vi "Prev_DaQ_QMH.vi"(8 "Error In":errorcluster, 11 "Queue In":refnum<queue>) -> (0 "Error Out":errorcluster, 1 "Message":variant, 2 "Instruction":T1=enum."Start DaQ", 3 "Queue Out":refnum<queue>)   [LabVIEW 2021, in "Queues.lvlib"]
doc: "This subVI is used to preveiew the DaQ QMH queue elements"
uses:
  Queues.lvlib
  Tipski Definicii/QMH_Daq_States.ctl
panel:
  # "Input"
  # "Output"
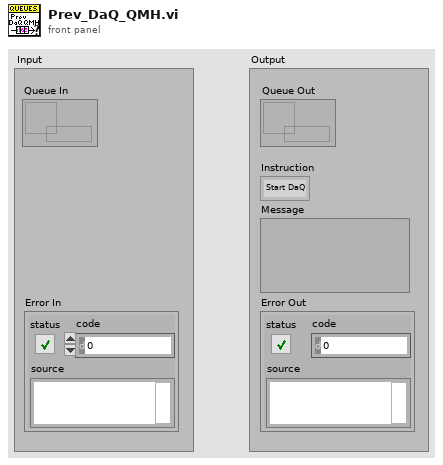
[diagram p1: front panel]
types:
  T1 = typedef "QMH_Daq_States.ctl" = enum16{"Idle", "Start DaQ", "DaQ", "Generate Message", "Stop DaQ", "End"}
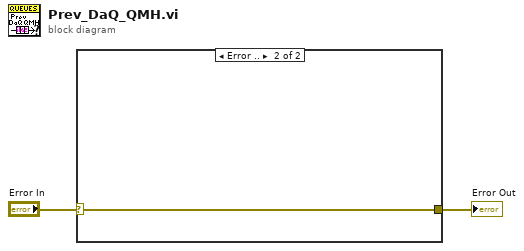
[diagram p0: block diagram]
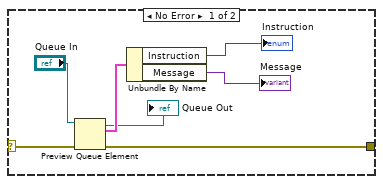
[diagram p2: hidden frame]
diagram:
  n1 = case shown="Error .." "Error In" {
    selector: "Error In" -> [w9 w10]
    tunnel: [w4 w10] -> w1
    frame No Error {
      n2 = Preview Queue Element(queue="Queue In", error in (no error)=w9) -> (queue out=→"Queue Out":refnum<queue>, element=w7:cluster{"Instruction":T1, "Message":variant}, error out=w4:errorcluster)  [unwired: 1 in, 1 out]
      n3 = Unbundle By Name(w7) -> ("Instruction"=→"Instruction":T1, "Message"=→"Message":variant)
    }
    frame Error {
    }
  }
  "Error Out" <- w1
